vi "Lookup API by Identity.vi"(8 "error in (no error)":errorcluster, 10 "Identity":refnum<class "Identity.lvclass">, 11 "VolatusHandler in":refnum<class "VolatusHandler.lvclass">) -> (0 "error out":errorcluster, 3 "VolatusHandler out":refnum<class "VolatusHandler.lvclass">)   [LabVIEW 2020, in "Volatus.lvlib" / "VolatusHandler.lvclass"]
uses:
  VolatusHandler.lvclass
  Identity/Identity.lvclass
  lv-promises/Promises/Promise/Promise.lvclass
panel:
  in  "Promise":refnum<class "Promise.lvclass">
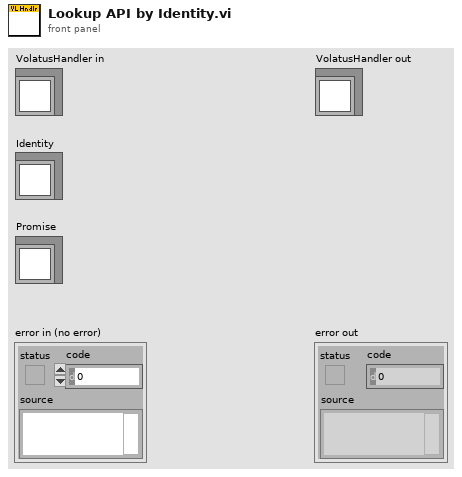
[diagram p1: front panel]
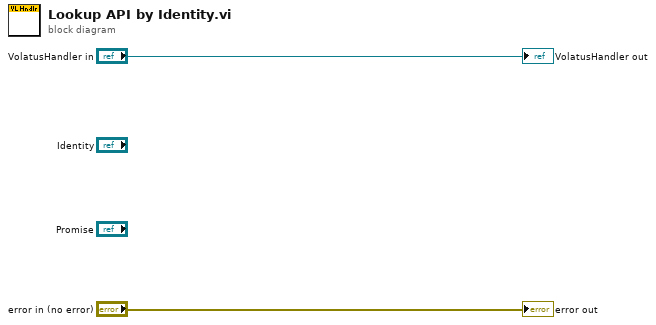
[diagram p0: block diagram]
diagram:
  "error out" <- "error in (no error)"
  "VolatusHandler out" <- "VolatusHandler in"
